vi "find_side_points.vi"(9 "corner":dbl[][](array[numeric]), 10 "X  coords array":dbl[](array[numeric]), 11 "Y coords array":dbl[](array[numeric])) -> (3 "side of clusters":cluster{"Array out":dbl[][]}[](array[cluster]))   [LabVIEW 2017]
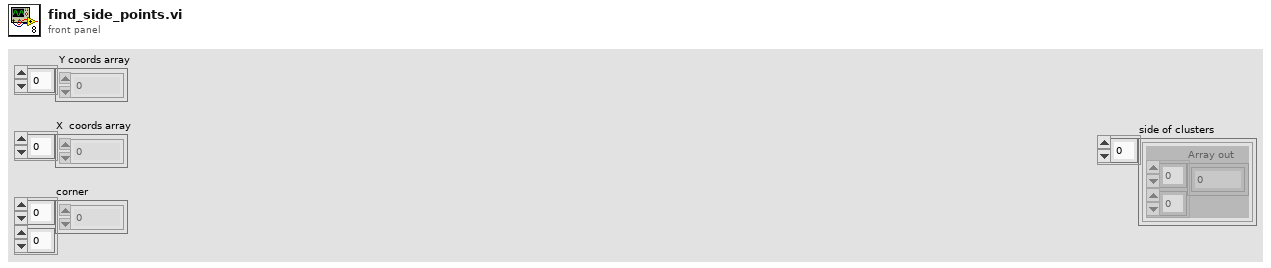
[diagram p1: front panel]
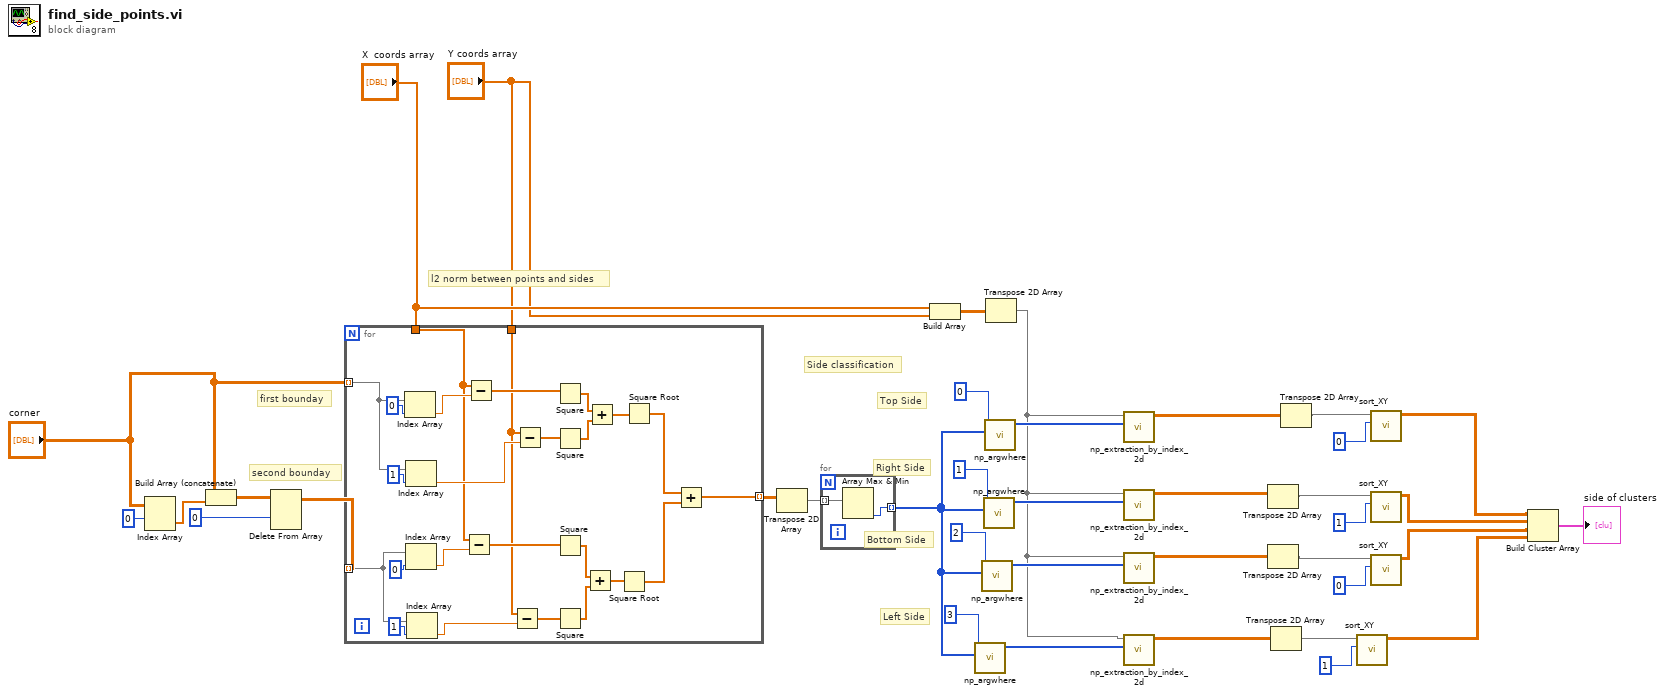
[diagram p0: block diagram]
diagram:
  # "Top Side"
  # "Left Side"
  # "Bottom Side"
  # "Right Side"
  # "l2 norm between points and sides"
  # "Side classification"
  # "first bounday"
  # "second bounday"
  n1 = Index Array "Index Array"(array="corner", index (row)=0 ("disabled index (col)")) -> (element=w24:dbl[])  [unwired: 1 in]
  n2 = Build Array (concatenate)("corner", w24) -> (w25:dbl[][])
  n3 = Delete From Array(array=w25, index (row)=0) -> (array with subset deleted=w28:dbl[][])  [unwired: 2 in, 1 out]
  n4 = for {
    tunnel: "corner" -> [w61] mode=indexing
    tunnel: w28 -> [w57] mode=indexing
    tunnel: [w41] -> w29 mode=indexing
    tunnel: "X  coords array" -> [w40]
    tunnel: "Y coords array" -> [w39]
    n5 = Index Array(array=w61, index=0) -> (element=w60:dbl)
    n6 = Index Array(array=w61, index=1) -> (element=w56:dbl)
    n7 = Index Array(array=w57, index=0) -> (element=w55:dbl)
    n8 = Index Array(array=w57, index=1) -> (element=w54:dbl)
    n9 = Subtract(x=w40, y=w55) -> (x-y=w51:dbl[])
    n10 = Subtract(x=w40, y=w60) -> (x-y=w53:dbl[])
    n11 = Subtract(x=w39, y=w54) -> (x-y=w50:dbl[])
    n12 = Subtract(x=w39, y=w56) -> (x-y=w52:dbl[])
    n13 = Square(x=w53) -> (x^2=w49:dbl[])
    n14 = Square(x=w52) -> (x^2=w48:dbl[])
    n15 = Square(x=w51) -> (x^2=w47:dbl[])
    n16 = Square(x=w50) -> (x^2=w46:dbl[])
    n17 = Add(x=w47, y=w46) -> (x+y=w44:dbl[])
    n18 = Add(x=w49, y=w48) -> (x+y=w45:dbl[])
    n19 = Square Root(x=w44) -> (sqrt(x)=w42:dbl[])
    n20 = Square Root(x=w45) -> (sqrt(x)=w43:dbl[])
    n21 = Add(x=w43, y=w42) -> (x+y=w41:dbl[])
  }
  n22 = Transpose 2D Array(2D array=w29) -> (transposed array=w30:dbl[][])
  n23 = for {
    tunnel: w30 -> [w65] mode=indexing
    tunnel: [w64] -> w38 mode=indexing
    n24 = Array Max & Min(array=w65) -> (min index (indices)=w64:i32)  [unwired: 3 out]
  }
  n25 = Build Array("X  coords array", "Y coords array") -> (w33:dbl[][])
  n26 = call "np_argwhere.vi"("Array in"=w38, "value"=3) -> ("index"=w10:i32[])  [unwired: 9 in]
  n27 = call "np_argwhere.vi"("Array in"=w38, "value"=2) -> ("index"=w11:i32[])  [unwired: 9 in]
  n28 = call "np_argwhere.vi"("Array in"=w38, "value"=1) -> ("index"=w12:i32[])  [unwired: 9 in]
  n29 = call "np_argwhere.vi"("Array in"=w38, "value"=0) -> ("index"=w14:i32[])  [unwired: 9 in]
  n30 = Transpose 2D Array(2D array=w33) -> (transposed array=w6:dbl[][])
  n31 = call "np_extraction_by_index_2d.vi"("index array"=w14, "Array in"=w6) -> ("Array out"=w13:dbl[][])  [unwired: 9 in]
  n32 = call "np_extraction_by_index_2d.vi"("index array"=w12, "Array in"=w6) -> ("Array out"=w9:dbl[][])  [unwired: 9 in]
  n33 = call "np_extraction_by_index_2d.vi"("index array"=w11, "Array in"=w6) -> ("Array out"=w8:dbl[][])  [unwired: 9 in]
  n34 = call "np_extraction_by_index_2d.vi"("index array"=w10, "Array in"=w6) -> ("Array out"=w7:dbl[][])  [unwired: 9 in]
  n35 = Transpose 2D Array(2D array=w9) -> (transposed array=w16:dbl[][])
  n36 = Transpose 2D Array(2D array=w8) -> (transposed array=w15:dbl[][])
  n37 = Transpose 2D Array(2D array=w7) -> (transposed array=w22:dbl[][])
  n38 = Transpose 2D Array(2D array=w13) -> (transposed array=w17:dbl[][])
  n39 = call "sort_XY.vi"("sort axis"=1 ("index (row)"), "Array in"=w22) -> ("Array out"=w2:dbl[][])  [unwired: 9 in]
  n40 = call "sort_XY.vi"("sort axis"=0 ("index (row)"), "Array in"=w17) -> ("Array out"=w5:dbl[][])  [unwired: 9 in]
  n41 = call "sort_XY.vi"("sort axis"=1 ("index (row)"), "Array in"=w16) -> ("Array out"=w4:dbl[][])  [unwired: 9 in]
  n42 = call "sort_XY.vi"("sort axis"=0 ("index (row)"), "Array in"=w15) -> ("Array out"=w3:dbl[][])  [unwired: 9 in]
  n43 = Build Cluster Array(w5, w4, w3, w2) -> (→"side of clusters":cluster{"Array out":dbl[][]}[])
